vi "Regexp Filtering.vi"() -> ()   [LabVIEW 2012]
uses:
  <userlib>/_OpenG.lib/array/array.llb/Filter 1D Array (String)__ogtk.vi
  <userlib>/_LAVAcr/OpenG Array XNodes/OpenG Filter Array/OpenG FilterArray.xnode
panel:
  out "Same?":bool
  out "XNode Time":dbl format="%#_6ps"
  out "OpenG Time":dbl format="%#_6ps"
  out "XNode Filtered Indices":i32[](array[numeric])
  out "XNode Filters":string[](array[string])
  out "OpenG Array Filter Indices":i32[](array[numeric])
  out "OpenG Array Filter":string[](array[string])
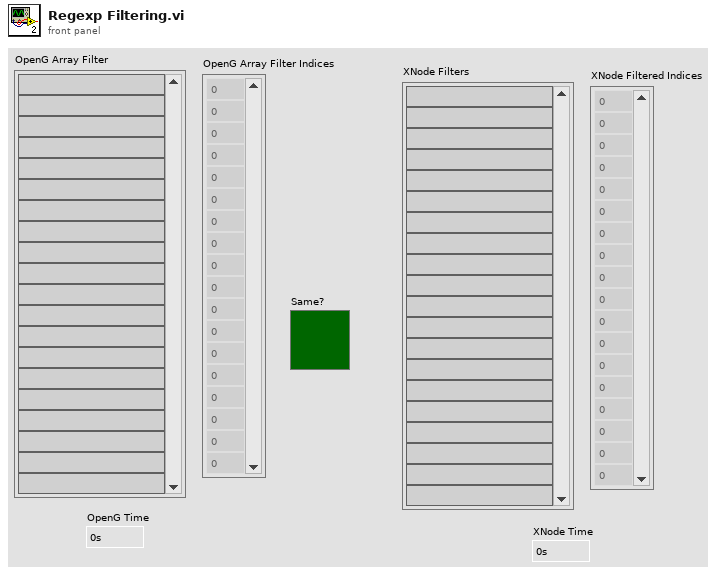
[diagram p1: front panel]
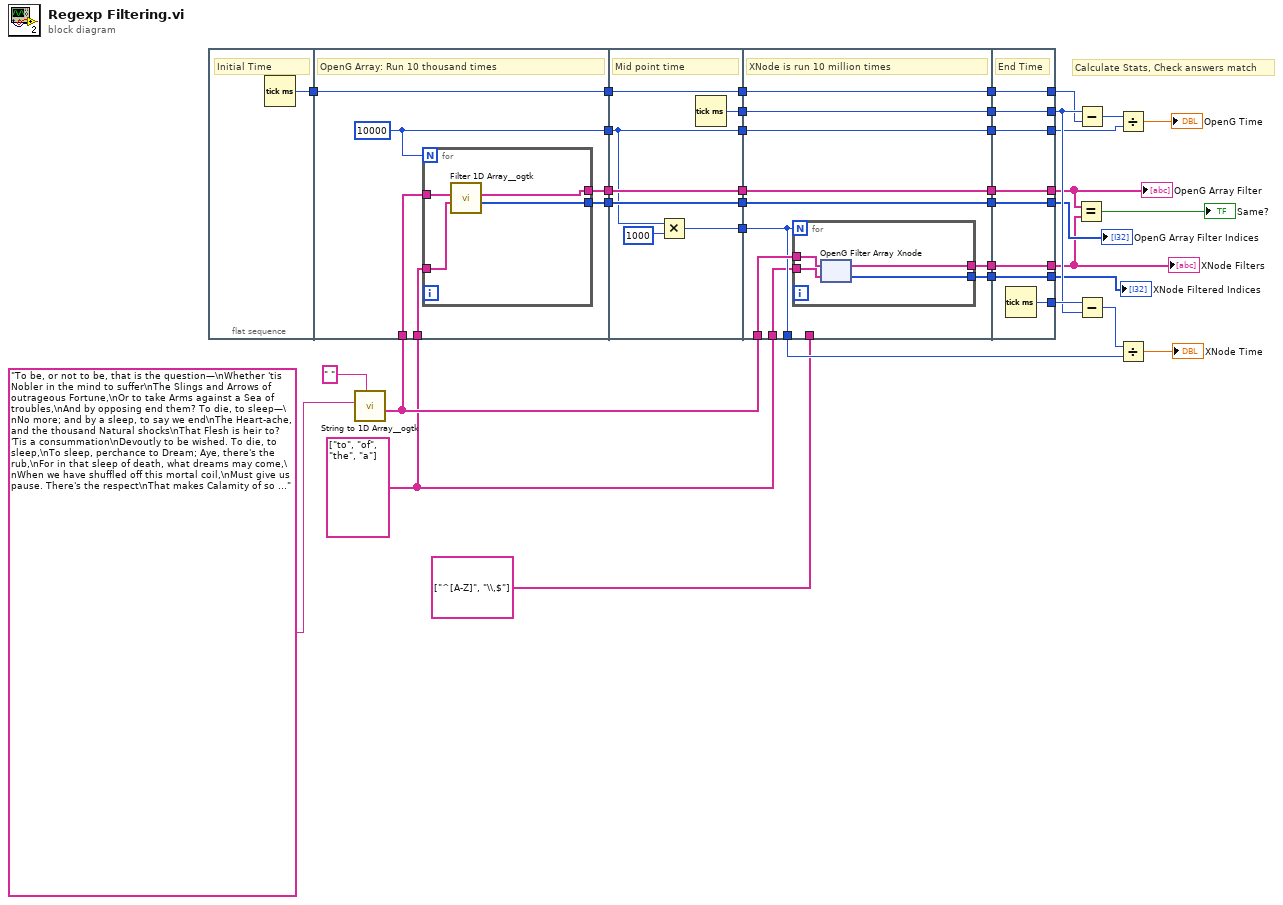
[diagram p0: block diagram]
diagram:
  w34 = string[] ["to", "of", "the", "a"]
  # "Calculate Stats, Check answers match"
  n1 = flat-sequence {
    tunnel: [w38] -> w28
    tunnel: w35 -> [w44]
    tunnel: w34 -> [w43]
    tunnel: [w42] -> w29
    tunnel: w28 -> [w42]
    tunnel: [w41] -> w20
    tunnel: [w40] -> w16
    tunnel: [w39] -> w13
    tunnel: [w55] -> w32
    tunnel: [w54] -> w30
    tunnel: w29 -> [w54]
    tunnel: w20 -> [w51]
    tunnel: [w51] -> w19
    tunnel: w16 -> [w53]
    tunnel: [w53] -> w15
    tunnel: w13 -> [w52]
    tunnel: [w52] -> w12
    tunnel: [w49] -> w3
    tunnel: w35 -> [w65]
    tunnel: w34 -> [w56]
    tunnel: [w64] -> w33
    tunnel: w32 -> [w64]
    tunnel: [w63] -> w31
    tunnel: w30 -> [w63]
    tunnel: w19 -> [w62]
    tunnel: [w62] -> w18
    tunnel: w15 -> [w61]
    tunnel: [w61] -> w14
    tunnel: w12 -> [w60]
    tunnel: [w60] -> w11
    tunnel: [w59] -> w9
    tunnel: [w58] -> w8
    tunnel: w3 -> [w57]
    tunnel: [w57] -> w2
    tunnel: string[] ["^[A-Z]", "\\,$"] -> [_]
    tunnel: [w116] -> w27
    tunnel: [w115] -> w26
    tunnel: w33 -> [w115]
    tunnel: [w114] -> w25
    tunnel: w31 -> [w114]
    tunnel: w18 -> [w113]
    tunnel: [w113] -> w17
    tunnel: w14 -> [w112]
    tunnel: [w112] -> w6
    tunnel: w11 -> [w111]
    tunnel: [w111] -> w10
    tunnel: w9 -> [w110]
    tunnel: [w110] -> w5
    tunnel: w8 -> [w109]
    tunnel: [w109] -> w7
    frame #0 {
      # "Initial Time"
      n2 = Tick Count (ms)() -> (millisecond timer value=w38:u32)
    }
    frame #1 {
      w41 = 10000
      # "OpenG Array: Run 10 thousand times"
      n3 = for {
        N: w41 -> [_]
        tunnel: [w48] -> w40
        tunnel: w44 -> [w47]
        tunnel: [w46] -> w39
        tunnel: w43 -> [w45]
        n4 = call-poly <userlib>:"Filter 1D Array__ogtk.vi"("items to filter"=w45, "array"=w47) -> ("filtered item indices"=w46:i32[], "filtered array"=w48:string[])  [unwired: 4 in]
      }
    }
    frame #2 {
      # "Mid point time"
      n5 = Multiply(x=w51, y=1000) -> (x*y=w49:i32)
      n6 = Tick Count (ms)() -> (millisecond timer value=w55:u32)
    }
    frame #3 {
      # "XNode is run 10 million times"
      n7 = for {
        N: w57 -> [_]
        tunnel: w65 -> [w69]
        tunnel: w56 -> [w68]
        tunnel: [w67] -> w59
        tunnel: [w66] -> w58
        n8 = xnode "OpenG Filter Array Xnode"("array"=w69, "items to filter"=w68) -> ("filtered items"=w67:string[], "filtered item indices"=w66:i32[])
      }
    }
    frame #4 {
      # "End Time"
      n9 = Tick Count (ms)() -> (millisecond timer value=w116:u32)
    }
  }
  n10 = call <userlib>:"String to 1D Array__ogtk.vi"("delimiter (Tab)"=" ", "string"="To be, or not to be, that is the question—\nWhether 'tis Nobler in the mind to suffer\nThe Slings and Arrows of outrageous Fortune,\nOr to take Arms against a Sea of troubles,\nAnd by opposing end them? To die, to sleep—\nNo more; and by a sleep, to say we end\nThe Heart-ache, and the thousand Natural shocks\nThat Flesh is heir to? 'Tis a consummation\nDevoutly to be wished. To die, to sleep,\nTo sleep, perchance to Dream; Aye, there's the rub,\nFor in that sleep of death, what dreams may come,\nWhen we have shuffled off this mortal coil,\nMust give us pause. There's the respect\nThat makes Calamity of so long life:\nFor who would bear the Whips and Scorns of time,\nThe Oppressor's wrong, the proud man's Contumely,\nThe pangs of despised Love, the Law’s delay,\nThe insolence of Office, and the Spurns\nThat patient merit of the unworthy takes,\nWhen he himself might his Quietus make\nWith a bare Bodkin? Who would these Fardels bear,\nTo grunt and sweat under a weary life,\nBut that the dread of something after death,\nThe undiscovered Country, from whose bourn\nNo Traveler returns, Puzzles the will,\nAnd makes us rather bear those ills we have,\nThan fly to others that we know not of.\nThus Conscience does make Cowards of us all,\nAnd thus the Native hue of Resolution\nIs sicklied o'er, with the pale cast of Thought,\nAnd enterprises of great pitch and moment,\nWith this regard their Currents turn awry,\nAnd lose the name of Action. Soft you now,\nThe fair Ophelia. Nymph, in all thy Orisons\nBe thou all my sins remembered.") -> ("Array of Strings"=w35:string[])  [unwired: 9 in]
  n11 = Equal?(x=w6, y=w5) -> (x = y?=→"Same?":bool)
  n12 = Subtract(x=w26, y=w25) -> (x-y=w24:u32)
  n13 = Subtract(x=w27, y=w26) -> (x-y=w23:u32)
  n14 = Divide(x=w24, y=w17) -> (x/y=→"OpenG Time":dbl)
  n15 = Divide(x=w23, y=w2) -> (x/y=→"XNode Time":dbl)
  "OpenG Array Filter" <- w6
  "OpenG Array Filter Indices" <- w10
  "XNode Filters" <- w5
  "XNode Filtered Indices" <- w7
